vi "Read Attributes.vi"(11 "A_msg Msg":refnum<class "A_msg Msg.lvclass">) -> (2 "Payload":cluster{"Status":string})   [LabVIEW 2025, in "A_Actor.lvlib" / "A_msg Msg.lvclass"]
uses:
  A_msg Msg.lvclass
  A_msg Msg.lvclass/A_msg Msg.ctl
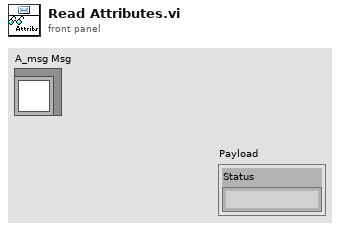
[diagram p1: front panel]
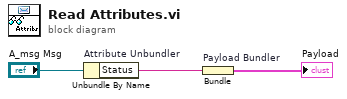
[diagram p0: block diagram]
diagram:
  n1 = Unbundle By Name "Attribute Unbundler"("A_msg Msg") -> ("Status"=w1:string)
  n2 = Bundle "Payload Bundler"("Status"=w1) -> (→"Payload":cluster{"Status":string})  [unwired: 1 in]
